vi "lock-in amplifier SR830.vi"(10 "Integration time (ms)":dbl, 11 "Connection":refnum<visa-resource-name>) -> (3 "mean":dbl format="%0.2f")   [LabVIEW 2024]
uses:
  <vilib>/Analysis/baseanly.llb/Mean (DBL).vi
  <vilib>/Analysis/NI_AALBase.lvlib
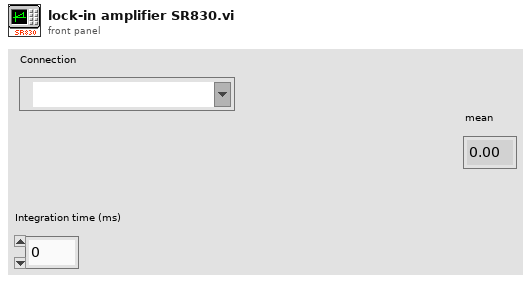
[diagram p1: front panel]
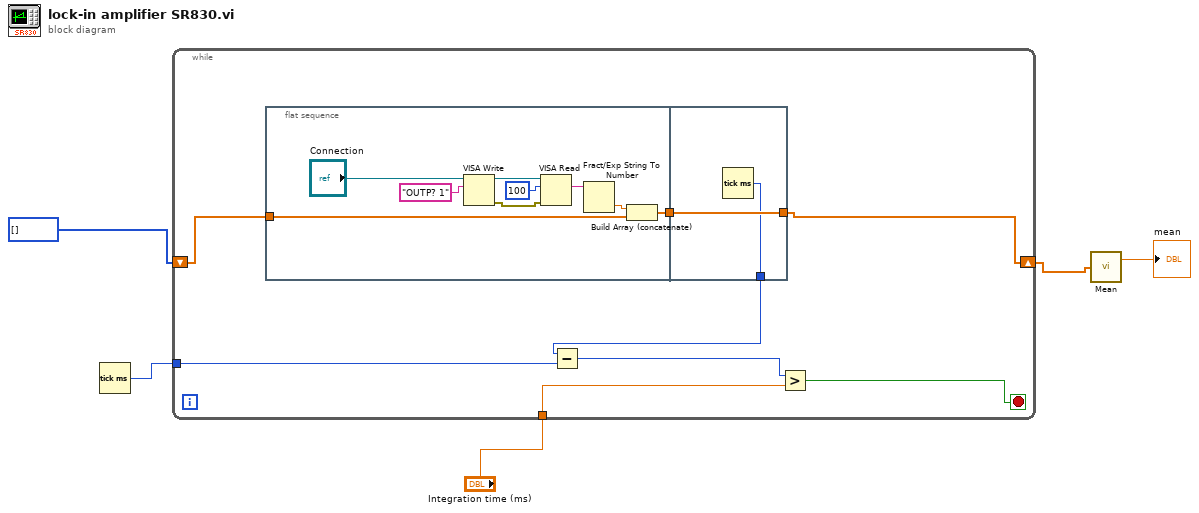
[diagram p0: block diagram]
diagram:
  n1 = Tick Count (ms)() -> (millisecond timer value=w4:u32)
  n2 = while {
    shift-right: [w13] -> w2
    shift-left: i32[] [] -> [w12]
    tunnel: w4 -> [w9]
    tunnel: "Integration time (ms)" -> [w6]
    stop <- w7 stop-if-true
    n3 = flat-sequence {
      tunnel: w12 -> [w15]
      tunnel: [w16] -> w11
      tunnel: [w24] -> w13
      tunnel: w11 -> [w24]
      tunnel: [w23] -> w10
      frame #0 {
        n4 = VISA Write(VISA resource name="Connection", write buffer="OUTP? 1") -> (VISA resource name out=w22:refnum<visa-resource-name>, error out=w14:errorcluster)  [unwired: 1 in, 1 out]
        n5 = VISA Read(VISA resource name=w22, byte count=u32 100, error in (no error)=w14) -> (read buffer=w18:string)  [unwired: 3 out]
        n6 = Fract/Exp String To Number(string=w18) -> (number=w17:dbl)  [unwired: 3 in, 1 out]
        n7 = Build Array (concatenate)(w17, w15) -> (w16:dbl[])
      }
      frame #1 {
        n8 = Tick Count (ms)() -> (millisecond timer value=w23:u32)
      }
    }
    n9 = Subtract(x=w10, y=w9) -> (x-y=w8:u32)
    n10 = Greater?(x=w8, y=w6) -> (0:w7:bool)
  }
  n11 = call-poly <vilib>:"Mean.vi"("X"=w2) -> ("mean"=→"mean":dbl)  [unwired: 1 out]
